vi "WPI_UtilitiesFRC SendMessageToConsole.vi"(0 "Message":string, 11 "error in (no error)":errorcluster) -> (15 "error out":errorcluster)   [LabVIEW 2017]
doc: "Appends the string message to the console and DS log..\n\nThis software is licensed. Open the labview\\readme\\WPI Robotics Library Open Source License.txt file for more information."
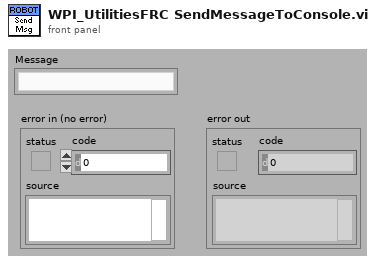
[diagram p1: front panel]
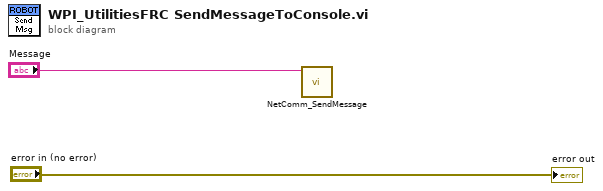
[diagram p0: block diagram]
diagram:
  n1 = call <vilib>:"NetComm_SendMessage.vi"("Message"="Message") -> ()  [unwired: 11 in]
  "error out" <- "error in (no error)"
